vi "Error Query.vi"(8 "error in":errorcluster, 11 "VISA resource in":refnum<visa-resource-name>) -> (0 "error out":errorcluster, 1 "Error Message":string, 2 "Error Code":i32[](array[numeric]), 3 "VISA resource out":refnum<visa-resource-name>)   [LabVIEW 2019, in "Acopian.lvlib" / "Acopian.lvclass"]
uses:
  Library/Acopian.lvclass
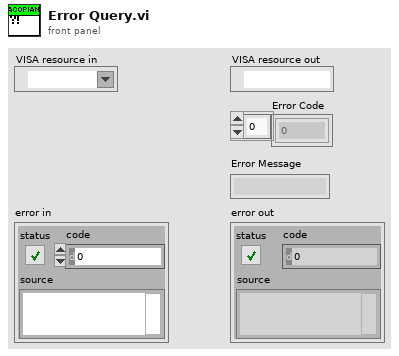
[diagram p1: front panel]
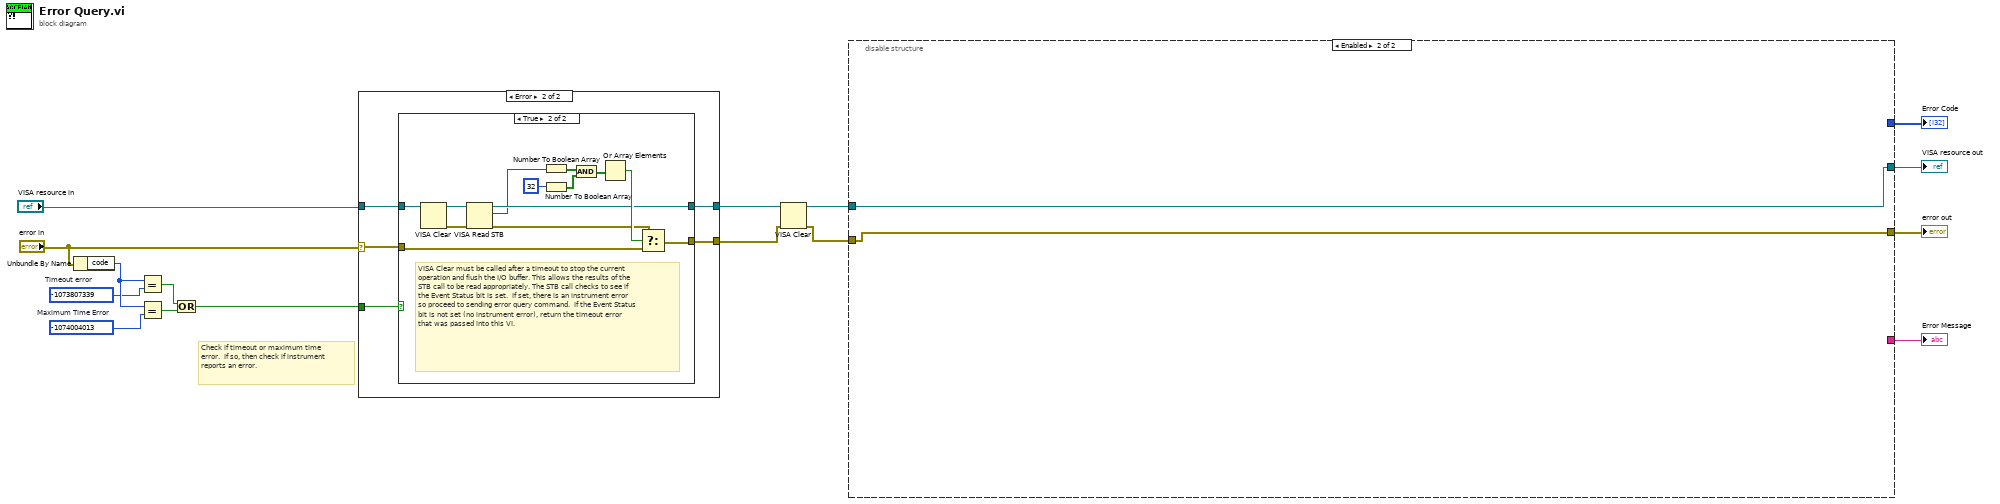
[diagram p0: block diagram]
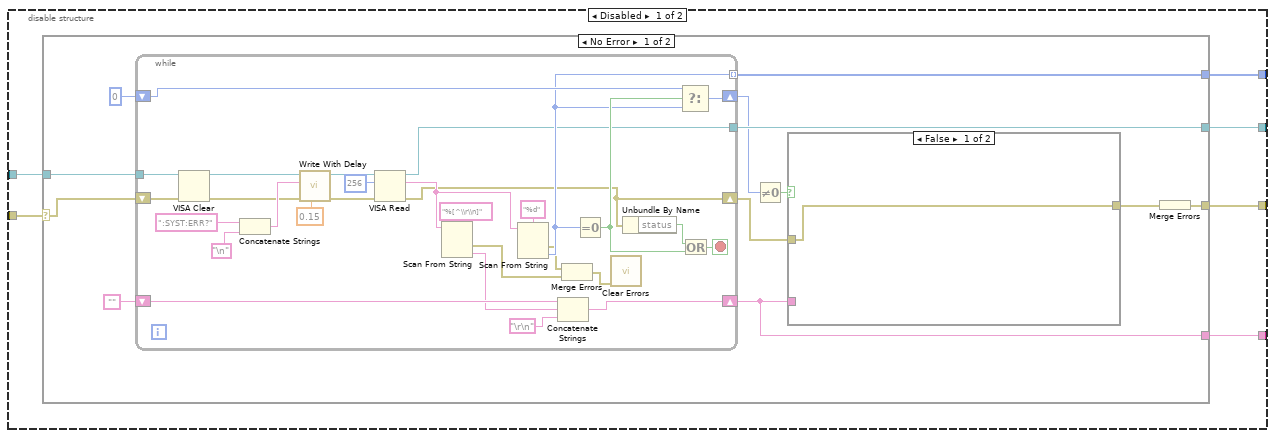
[diagram p2: hidden frame]
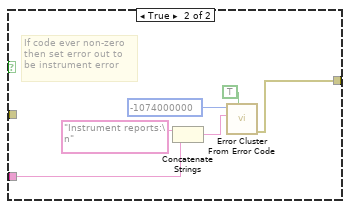
[diagram p3: hidden frame]
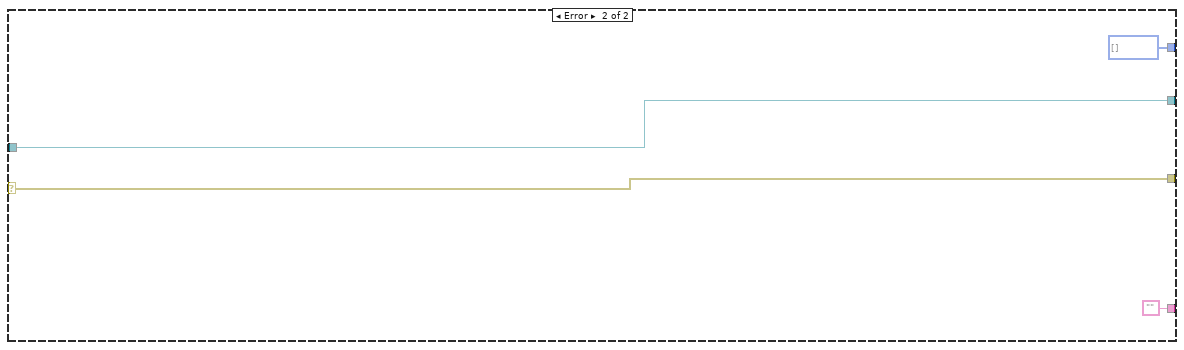
[diagram p4: hidden frame]
diagram:
  w13 = -1074004013  # Maximum Time Error
  w11 = -1073807339  # Timeout error
  # "Check if timeout or maximum time error.  If so, then check if instrument reports an error."
  n1 = Unbundle By Name("error in") -> ("code"=w12:i32)
  n2 = Equal?(x=w12, y=w11) -> (x = y?=w15:bool)
  n3 = Equal?(x=w12, y=w13) -> (x = y?=w14:bool)
  n4 = Or(x=w15, y=w14) -> (x .or. y?=w16:bool)
  n5 = case shown="Error" "error in" {
    selector: "error in" -> [w17 w21]
    tunnel: "VISA resource in" -> [w18 w23]
    tunnel: [w18 w22] -> w4
    tunnel: [w17 w20] -> w2
    tunnel: w16 -> [_ w19]
    frame No Error {
    }
    frame Error {
      n6 = case shown="True" w19 {
        tunnel: w23 -> [w25 w31]
        tunnel: [w25 w28] -> w22
        tunnel: w21 -> [w24 w34]
        tunnel: [w24 w33] -> w20
        frame False {
          # "Error code not a timeout, so best to pass on to user."
        }
        frame True {
          # "VISA Clear must be called after a timeout to stop the current operation and flush the I/O buffer. This allows the results of the  STB call to be read appropriately. The STB call checks to see if the Event Status bit is set.  If set, there is an instrument error so proceed to sending error query command.  If the Event Status bit is not set (no instrument error), return the timeout error that was passed into this VI."
          n7 = VISA Clear(VISA resource name=w31) -> (VISA resource name out=w30:refnum<visa-resource-name>, error out=w29:errorcluster)  [unwired: 1 in]
          n8 = VISA Read STB(8:w29, 11:w30) -> (0:w27:errorcluster, 2:w26:u16, 3:w28:refnum<visa-resource-name>)
          n9 = Number To Boolean Array(number=w26) -> (Boolean array=w35:bool[])
          n10 = Number To Boolean Array(number=32) -> (Boolean array=w37:bool[])
          n11 = And(x=w35, y=w37) -> (x .and. y?=w36:bool[])
          n12 = Or Array Elements(Boolean array=w36) -> (logical OR=w32:bool)
          n13 = Select(t=w27, s=w32, f=w34) -> (s? t:f=w33:errorcluster)
        }
      }
    }
  }
  n14 = VISA Clear(VISA resource name=w4, error in (no error)=w2) -> (VISA resource name out=w3:refnum<visa-resource-name>, error out=w1:errorcluster)
  n15 = disable-structure shown="Enabled" {
    disable-tunnel: [w44 w97] -> w8
    disable-tunnel: [w43 w98] -> w7
    disable-tunnel: [w42 _] -> w6
    disable-tunnel: [w41 _] -> w5
    disable-tunnel: w3 -> [w40 w98]
    disable-tunnel: w1 -> [w39 w97]
    frame Disabled {
      n16 = case shown="No Error" w39 {
        selector: w39 -> [w45 w93]
        tunnel: [w56 w96] -> w43
        tunnel: w40 -> [w55 w96]
        tunnel: [w53 w93] -> w44
        tunnel: [w48 ""] -> w41
        tunnel: [w47 i32[] []] -> w42
        frame No Error {
          n17 = while {
            tunnel: [w76] -> w56
            tunnel: w55 -> [w92]
            shift-right: [w84] -> w48
            shift-left: "" -> [w86]
            shift-right: [w82] -> w49
            shift-left: 0 -> [w83]
            shift-right: [w68] -> w46
            shift-left: w45 -> [w66]
            tunnel: [w77] -> w47 mode=indexing
            stop <- w88 stop-if-true
            n18 = VISA Clear(VISA resource name=w92, error in (no error)=w66) -> (VISA resource name out=w67:refnum<visa-resource-name>, error out=w65:errorcluster)
            n19 = Concatenate Strings(":SYST:ERR?" ("Error Query Command"), "\n") -> (w72:string)
            n20 = call "Write With Delay.vi"("Delay Time (s)"=0.15, "error in"=w65, "write buffer"=w72, "VISA resource name"=w67) -> ("error out"=w89:errorcluster, "VISA resource name out"=w91:refnum<visa-resource-name>)  [unwired: 6 in]
            n21 = VISA Read(VISA resource name=w91, byte count=u32 256 ("Bytes"), error in (no error)=w89) -> (VISA resource name out=w76:refnum<visa-resource-name>, read buffer=w75:string, error out=w68:errorcluster)  [unwired: 1 out]
            n22 = Scan From String(format string="%[^\\r\\n]", input string=w75) -> (error out=w69:errorcluster, output 1=w79:string)  [unwired: 3 in, 2 out]
            n23 = Scan From String(format string="%d", input string=w75) -> (error out=w70:errorcluster, output 1=w77:i32)  [unwired: 3 in, 2 out]
            n24 = Concatenate Strings(w86, w79, "\r\n") -> (w84:string)
            n25 = Merge Errors(w70, w69) -> (w71:errorcluster)
            n26 = Equal To 0?(x=w77) -> (x = 0?=w80:bool)
            n27 = call <vilib>:"Clear Errors.vi"("error in (no error)"=w71) -> ()  [unwired: 5 in, 2 out]
            n28 = Unbundle By Name(w68) -> ("status"=w81:bool)
            n29 = Select(t=w83, s=w80, f=w77) -> (s? t:f=w82:i32)
            n30 = Or(x=w81, y=w80) -> (x .or. y?=w88:bool)
          }
          n31 = Not Equal To 0?(x=w49) -> (x != 0?=w51:bool)
          n32 = case shown="False" w51 {
            tunnel: w48 -> [_ w62]
            tunnel: [w57 w58] -> w50
            tunnel: w46 -> [w57 _]
            frame False {
            }
            frame True {
              # "If code ever non-zero\nthen set error out to\nbe instrument error"
              n33 = Concatenate Strings("Instrument reports:\n" ("Source"), w62) -> (w59:string)
              n34 = call <vilib>:"Error Cluster From Error Code.vi"("show call chain? (False)"=TRUE, "error message (\"\")"=w59, "error code (0)"=-1074000000 ("Code")) -> ("error out"=w58:errorcluster)  [unwired: 6 in]
            }
          }
          n35 = Merge Errors(w50) -> (w53:errorcluster)
        }
        frame Error {
        }
      }
    }
    frame Enabled {
    }
  }
  "VISA resource out" <- w7
  "error out" <- w8
  "Error Code" <- w6
  "Error Message" <- w5
